vi "Shutdown.vi"(8 "error in":errorcluster, 11 "Instrument in":refnum<class "Instrument.lvclass">) -> (0 "error out":errorcluster, 3 "Instrument out":refnum<class "Instrument.lvclass">)   [LabVIEW 2014, in "Instrument.lvclass"]
doc: "General Instrument shutdown procedures. Kill open queues."
uses:
  Instrument.lvclass
  Session APIs/Session Log/System Log.lvclass
  Session APIs/File Access/Config Data/Config Data.lvclass
  Instrument.lvclass/Instrument.ctl
  <userlib>/_Session Fwk/Session - Root.lvclass
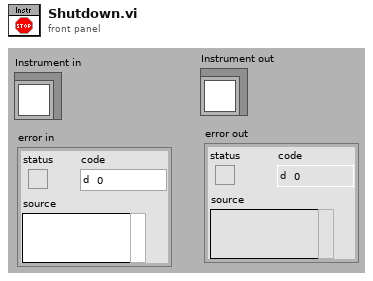
[diagram p1: front panel]
types:
  T1 = typedef "Session - Root.lvclass/Session Handle.ctl" = refnum<data-value>
  T2 = typedef "Config Data.lvclass/Config Session.ctl" = refnum<data-value>
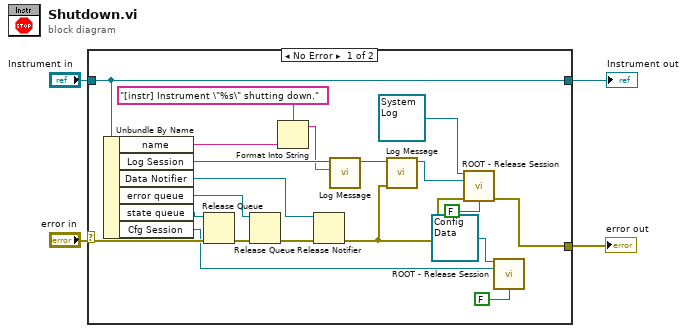
[diagram p0: block diagram]
diagram:
  n1 = case shown="No Error" "error in" {
    selector: "error in" -> [w22 w26]
    tunnel: [w19 w26] -> w3
    tunnel: [w24 w25] -> w1
    tunnel: "Instrument in" -> [w24 w25]
    frame No Error {
      n2 = Unbundle By Name(w24) -> ("name"=w13:string, "Log Session"=w16:T1, "Data Notifier"=w9:refnum<notifier>, "error queue"=w21:refnum<queue>, "state queue"=w23:refnum<queue>, "Cfg Session"=w6:T2)
      n3 = Release Queue(queue=w23, error in (no error)=w22) -> (error out=w20:errorcluster)  [unwired: 1 in, 2 out]
      n4 = Release Queue(queue=w21, error in (no error)=w20) -> (error out=w10:errorcluster)  [unwired: 1 in, 2 out]
      n5 = Format Into String(format string="[instr] Instrument \"%s\" shutting down.", w13) -> (resulting string=w11:string)  [unwired: 2 in, 1 out]
      n6 = Release Notifier(notifier=w9, error in (no error)=w10) -> (error out=w8:errorcluster)  [unwired: 1 in, 2 out]
      n7 = call "Log Message.vi"("MSG In"=w11, "session in"=w16) -> ("session out"=w15:T1)  [unwired: 8 in, 1 out]
      n8 = call "Log Message.vi"("error in"=w8, "session in"=w15) -> ("session out"=w14:T1)  [unwired: 8 in, 1 out]
      n9 = call <userlib>:"ROOT - Release Session.vi"("OBJ - Session in"=refnum<class "System Log.lvclass"> refnum ("Sys Log"), "Session Handle in"=w14, "error in (no error)"=w8, "force destroy? (F)"=FALSE) -> ("error out"=w19:errorcluster)  [unwired: 10 in, 1 out]
      n10 = call <userlib>:"ROOT - Release Session.vi"("OBJ - Session in"=refnum<class "Config Data.lvclass"> refnum ("Config Data"), "Session Handle in"=w6, "force destroy? (F)"=FALSE) -> ()  [unwired: 11 in, 2 out]
    }
    frame Error {
    }
  }
  "error out" <- w3
  "Instrument out" <- w1
